vi "Return_Data.vi"(8 "error in (no error)":errorcluster caption="entrée d'erreur (pas d'erreur)", 11 "Class DIO en entrée":refnum<class "Class Instrument Ana.lvclass">) -> (0 "error out":errorcluster caption="sortie d'erreur", 2 "Data_Json":string, 3 "Class DIO en Sortie":refnum<class "Class Instrument Ana.lvclass">)   [LabVIEW 2020, in "Library Instrument & Equipement.lvlib" / "Library Instruments.lvlib" / "Class Instrument Ana.lvclass"]
uses:
  Class Instrument Ana.lvclass
  Class Instrument Ana.lvclass/Class Instrument Ana.ctl
  JSON API/Variant JSON/Variant to JSON.vi
  JSON API/JSON Value/Get Item by name array.vi
  JSON API/JSON Value/JSON Value.lvclass
  JSON API/Get Polymorphic/JSON GetSet.lvlib
  JSON API/Variant JSON/Variant JSON.lvlib
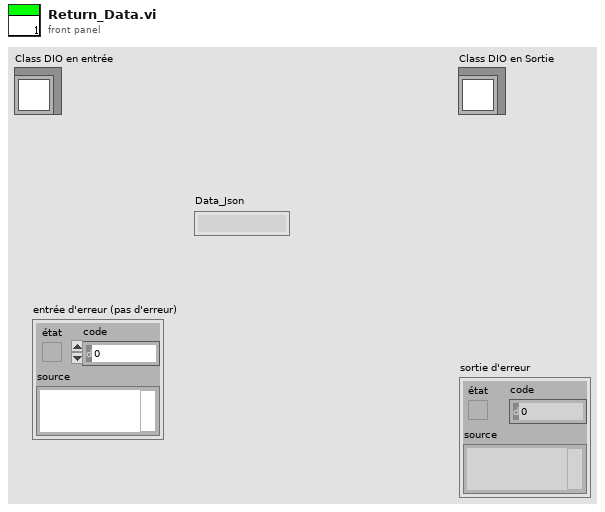
[diagram p1: front panel]
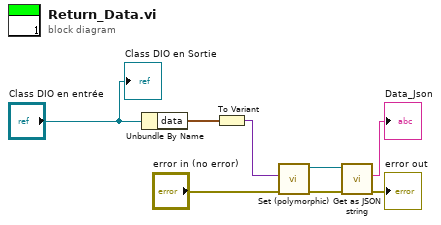
[diagram p0: block diagram]
diagram:
  n1 = Unbundle By Name("Class DIO en entrée") -> ("data"=w3:waveform(dbl)[])
  n2 = To Variant(anything=w3) -> (Variant=w8:variant)
  n3 = call-poly "Set (polymorphic).vi"("error in (no error)"="error in (no error)", "Variant"=w8) -> ("error out"=w6:errorcluster, "JSON Value out"=w7:refnum<class "JSON Value.lvclass">)  [unwired: 8 in]
  n4 = call "Get as JSON string.vi"("error in (no error)"=w6, "JSON Value in"=w7) -> ("error out"=→"error out":errorcluster, "<JSON>"=→"Data_Json":string)  [unwired: 8 in]
  "Class DIO en Sortie" <- "Class DIO en entrée"
